vi "Get DI historian from PGserver.vi"(4 "time_min":timestamp, 6 "time_max":timestamp, 9 "conninfo":T1={"host"="localhost", "port"="5432", "client_encoding"="WIN1251", "dbname"="data", "user"="postgres", "password"=""}, 10 "ParamColumns":string[](array[string])=["EPBP1_XQ01", "EPBP2_XQ01", "EPBP3_XQ01"], 11 "ParamTable":string="EP_XQ.1802") -> (0 "error out":errorcluster, 3 "Array":cluster{timestamp[], i16[]}[](array[cluster]))   [LabVIEW 2019, in "Inputs.lvlib"]
uses:
  Inputs.lvlib
  Database/PostgreSQL2LabVIEW/libpqlv/src/PQconnectdb.vi
  Database/PostgreSQL2LabVIEW/libpqlv/src/PQerrorMessage.vi
  Database/PostgreSQL2LabVIEW/libpqlv/src/PQstatus.vi
  <vilib>/dlg_ctls.llb/Space Constant.vi
  Database/PostgreSQL2LabVIEW/libpqlv/src/PQgetResult.vi
  Database/PostgreSQL2LabVIEW/libpqlv/src/PQclear.vi
  Database/PostgreSQL2LabVIEW/libpqUtility/src/PQfetchResultDataNotrans.vi
  Database/PostgreSQL2LabVIEW/libpqlv/src/PQresultErrorMessage.vi
  Database/PostgreSQL2LabVIEW/libpqlv/src/PQresultStatus.vi
  Database/PostgreSQL2LabVIEW/libpqlv/src/PQsendQuery.vi
  Database/PostgreSQL2LabVIEW/libpqlv/src/PQnfields.vi
  Database/PostgreSQL2LabVIEW/libpqlv/src/PQntuples.vi
  Database/PostgreSQL2LabVIEW/libpqlv/src/PQgetvalue.vi
  Database/PostgreSQL2LabVIEW/libpqUtility/libpqutility.lvlib
  Database/PostgreSQL2LabVIEW/libpqlv/libpqlv.lvlib
  Database/PostgreSQL.lvlib
panel:
  out "PQStatus":T2(ring)
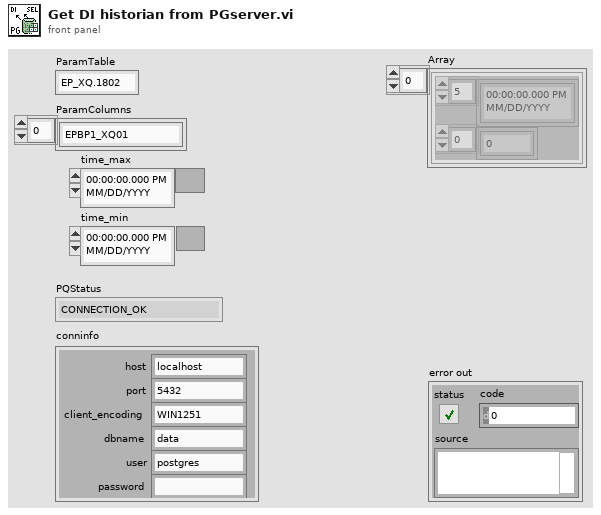
[diagram p1: front panel]
types:
  T1 = cluster{"host":string, "port":string, "client_encoding":string, "dbname":string, "user":string, "password":string}
  T2 = enum16{"CONNECTION_OK", "CONNECTION_BAD", "CONNECTION_STARTED", "CONNECTION_MADE", "CONNECTION_AWAITING_RESPONSE", "CONNECTION_AUTH_OK", "CONNECTION_SETENV", "CONNECTION_SSL_STARTUP", "CONNECTION_NEEDED"}
  T3 = enum32{"CONNECTION_OK", "CONNECTION_BAD", "CONNECTION_STARTED", "CONNECTION_MADE", "CONNECTION_AWAITING_RESPONSE", "CONNECTION_AUTH_OK", "CONNECTION_SETENV", "CONNECTION_SSL_STARTUP", "CONNECTION_NEEDED"}
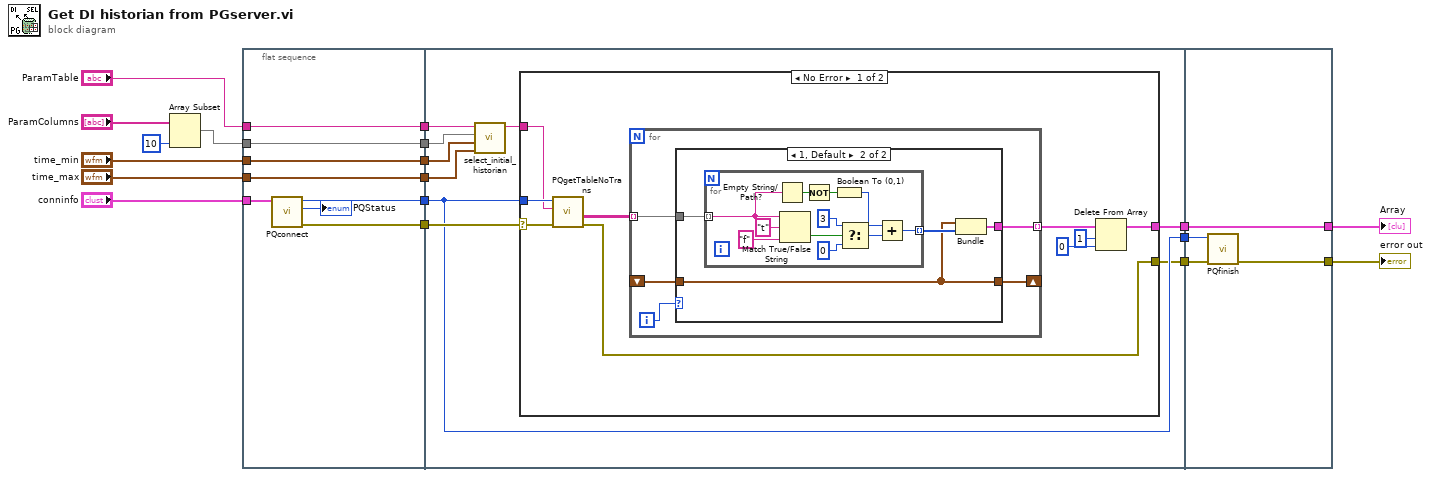
[diagram p0: block diagram]
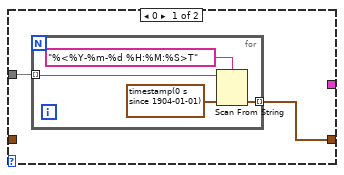
[diagram p2: hidden frame]
diagram:
  n1 = Array Subset(array="ParamColumns", length=10) -> (w3:string[])  [unwired: 1 in]
  n2 = flat-sequence {
    tunnel: [w26] -> w18
    tunnel: [w25] -> w17
    tunnel: [w21] -> w16
    tunnel: "ParamTable" -> [w26]
    tunnel: w3 -> [w25]
    tunnel: "conninfo" -> [w24]
    tunnel: [w23] -> w15
    tunnel: [w20] -> w9
    tunnel: "time_min" -> [w20]
    tunnel: [w19] -> w7
    tunnel: "time_max" -> [w19]
    tunnel: w18 -> [w32]
    tunnel: w17 -> [w31]
    tunnel: w16 -> [w34]
    tunnel: [w35] -> w14
    tunnel: w15 -> [w33]
    tunnel: [w33] -> w13
    tunnel: [w29] -> w10
    tunnel: w9 -> [w28]
    tunnel: w7 -> [w27]
    tunnel: [w75] -> w2
    tunnel: w14 -> [w75]
    tunnel: [w73] -> w1
    tunnel: w13 -> [w72]
    tunnel: w10 -> [w74]
    frame #0 {
      n3 = call "PQconnect.vi"("conninfo"=w24) -> ("error out"=w21:errorcluster, "PQStatus"=→"PQStatus":T3, "conn"=w23:u32)  [unwired: 8 in]
    }
    frame #1 {
      n4 = call "select_initial_historian.vi"("time_max"=w27, "time_min"=w28, "Column table"=w31, "table"=w32) -> ("parameters"=w30:string)  [unwired: 7 in]
      n5 = case shown="No Error" w34 {
        selector: w34 -> [w39 w71]
        tunnel: [w41 _] -> w35
        tunnel: w33 -> [w40 _]
        tunnel: w30 -> [w38 _]
        tunnel: [w36 w71] -> w29
        frame No Error {
          n6 = call "PQgetTableNoTrans.vi"("error in"=w39, "query"=w38, "conn"=w40) -> ("error out"=w36:errorcluster, "Data"=w37:string[][])  [unwired: 4 in, 3 out]
          n7 = for {
            tunnel: [w48] -> w44 mode=indexing
            tunnel: w37 -> [w49] mode=indexing
            shift-right: [w47] -> _
            shift-left: _ -> [w46]
            i -> [w45]
            n8 = case shown="1, Default" w45 {
              tunnel: [w51 w56] -> w47
              tunnel: w49 -> [w50 w59]
              tunnel: [_ w57] -> w48
              tunnel: w46 -> [_ w56]
              frame 0 {
                n9 = for {
                  tunnel: [w52] -> w51 mode=indexing
                  tunnel: w50 -> [w53] mode=indexing
                  n10 = Scan From String(format string="%<%Y-%m-%d %H:%M:%S>T" ("string"), input string=w53, default 1=timestamp(0 s since 1904-01-01) ("time stamp")) -> (output 1=w52:timestamp)  [unwired: 2 in, 3 out]
                }
              }
              frame 1, Default {
                n11 = for {
                  tunnel: w59 -> [w68] mode=indexing
                  tunnel: [w64] -> w58 mode=indexing
                  n12 = Empty String/Path?(string/path=w68) -> (empty?=w67:bool)
                  n13 = Match True/False String(2:"f" ("false string"), 3:"t" ("true string"), 4:w68) -> (0:w63:bool)  [unwired: 1 out]
                  n14 = Not(x=w67) -> (.not. x?=w66:bool)
                  n15 = Boolean To (0,1)(Boolean=w66) -> (0, 1=w65:i16)
                  n16 = Select(t=i16 3 ("0, 1"), s=w63, f=i16 0 ("0, 1")) -> (s? t:f=w60:i16)
                  n17 = Add(x=w65, y=w60) -> (x+y=w64:i16)
                }
                n18 = Bundle(w56, w58) -> (w57:cluster{timestamp[], i16[]})  [unwired: 1 in]
              }
            }
          }
          n19 = Delete From Array(array=w44, length=1, index=0) -> (array with subset deleted=w41:cluster{timestamp[], i16[]}[])  [unwired: 1 out]
        }
        frame Error {
        }
      }
    }
    frame #2 {
      n20 = call "PQfinish.vi"("error in (no error)"=w74, "conn"=w72) -> ("error out"=w73:errorcluster)  [unwired: 9 in]
    }
  }
  "Array" <- w2
  "error out" <- w1
